vi "main(Test DQMH modules).vi"() -> ()   [LabVIEW 2018, in "Application.lvlib"] (continued)
          frame condition #0 (active) {
            n3006 = Empty String/Path?(string/path=w7173) -> (empty?=w7175:bool)
            n3007 = Select(t="Quece timeout", s=w7175, f=w7173) -> (s? t:f=w7172:string)
            n3008 = call "string log (SubVI).vi"("state Name"=w7172) -> ()  [unwired: 9 in, 2 out]
          }
          frame condition #1 {
          }
        }
        n3009 = Bundle By Name(cluster=w7125, "command"="Apps.UI Update", "data"="E") -> (w7124:T9)
        n3010 = Bundle By Name(cluster=w7125, "command"="MEAS.AllRelaysOFF2") -> (w7117:T9)
        n3011 = Bundle By Name(cluster=w7125, "command"="Apps.WaitForEvent") -> (w7123:T9)
        n3012 = Build Array(w7124, w7117, w7123) -> (w7130:T9[])
        n3013 = for {
          tunnel: [w7163] -> w7136 mode=indexing
          shift-right: [w7164] -> w7138
          shift-left: w7131 -> [w7162]
          tunnel: w7130 -> [w7161] mode=indexing
          n3014 = Unbundle By Name(w7161) -> ("command"=w7160:string, "data"=w7159:variant)
          n3015 = call "App enquece.vi"("Priority Enquece"=TRUE, "command data"=w7159, "command"=w7160, "queue in"=w7162) -> ("error out"=w7163:errorcluster, "Queue out"=w7164:refnum<queue>)  [unwired: 6 in]
        }
        n3016 = call "FGV DRV stand.vi"() -> ("Sub-Test.DCV"=w7118:bool)  [unwired: 10 in, 1 out]
        n3017 = case shown="True" w7118 {
          tunnel: [w7149 w7151] -> w7120
          frame False {
            n3018 = Build Array("WaitFor", "MEAS.requestAC") -> (w7149:string[])
          }
          frame True {
            n3019 = Build Array("Test DRV 31", "Test DRV 32", "Test DRV 33", "Test DRV 34", "Test DRV 35", "WaitForE", "MEAS.requestAC") -> (w7151:string[])
          }
        }
        n3020 = Merge Errors(w7136) -> (w7129:errorcluster)
        n3021 = Reverse 1D Array(array=w7120) -> (reversed array=w7116:string[])
        n3022 = for {
          tunnel: w7116 -> [w7170] mode=indexing
          tunnel: [w7169] -> w7135 mode=indexing
          shift-right: [w7168] -> w7137
          shift-left: w7138 -> [w7171]
          tunnel: w7129 -> [w7167]
          n3023 = call "App enquece.vi"("Priority Enquece"=TRUE, "error in (no error)"=w7167, "command"=w7170, "queue in"=w7171) -> ("error out"=w7169:errorcluster, "Queue out"=w7168:refnum<queue>)  [unwired: 6 in]
        }
        n3024 = Initialize Array(FALSE ("element"), 6 ("dimension size")) -> (w7099:bool[])
        n3025 = Initialize Array(TRUE, 5 ("dimension size")) -> (w7098:bool[])
        n3026 = Merge Errors(w7135) -> (w7134:errorcluster)
        n3027 = Replace Array Subset(array=w7099, new element=w7098) -> (w7097:bool[])  [unwired: 1 in]
        n3028 = To Variant(anything=T3."mux10_1_channel6" ("mux10_1(x6)_encode")) -> (Variant=w7114:variant)
        n3029 = To Variant(anything=T4."demux1_10_channel6" ("demux1_10(x6)_encode")) -> (Variant=w7110:variant)
        n3030 = To Variant(anything=w7097) -> (Variant=w7106:variant)
        n3031 = Bundle By Name(cluster=w7103, "command"="MEAS.mux10-1", "data"=w7114) -> (w7109:T9)
        n3032 = Bundle By Name(cluster=w7103, "command"="MEAS.demux1-10", "data"=w7110) -> (w7108:T9)
        n3033 = Bundle By Name(cluster=w7103, "command"="MEAS.eMIC", "data"=w7106) -> (w7105:T9)
        n3034 = Build Array(w7109, w7108, w7105) -> (w7133:T9[])
        n3035 = Reverse 1D Array(array=w7133) -> (reversed array=w7132:T9[])
        n3036 = for {
          tunnel: w7132 -> [w7181] mode=indexing
          tunnel: [w7178] -> w7139 mode=indexing
          tunnel: w7134 -> [w7177]
          tunnel: w7137 -> [w7182]
          n3037 = Unbundle By Name(w7181) -> ("command"=w7180:string, "data"=w7179:variant)
          n3038 = call "App enquece.vi"("Priority Enquece"=TRUE, "error in (no error)"=w7177, "command data"=w7179, "command"=w7180, "queue in"=w7182) -> ("error out"=w7178:errorcluster)  [unwired: 5 in, 1 out]
        }
        n3039 = Merge Errors(w7142, w7139) -> (w7143:errorcluster)
      }
      frame "Test Channel 7E" {
        w7189 = T9 {"command"="", "data"=variant} ("element")
        w7212 = T9 {"command"="", "data"=variant} ("element")
        w7231 = 7  # DUT channel (1-10)
        n3040 = disable-structure shown="LOGGING==TRUE" {
          disable-tunnel: w7226 -> [w7259 _]
          frame condition #0 (active) {
            n3041 = Empty String/Path?(string/path=w7259) -> (empty?=w7261:bool)
            n3042 = Select(t="Quece timeout", s=w7261, f=w7259) -> (s? t:f=w7258:string)
            n3043 = call "string log (SubVI).vi"("state Name"=w7258) -> ()  [unwired: 9 in, 2 out]
          }
          frame condition #1 {
          }
        }
        n3044 = Bundle By Name(cluster=w7212, "command"="Apps.UI Update", "data"="E") -> (w7211:T9)
        n3045 = Bundle By Name(cluster=w7212, "command"="MEAS.AllRelaysOFF2") -> (w7204:T9)
        n3046 = Bundle By Name(cluster=w7212, "command"="Apps.WaitForEvent") -> (w7210:T9)
        n3047 = Build Array(w7211, w7204, w7210) -> (w7202:T9[])
        n3048 = for {
          tunnel: [w7249] -> w7222 mode=indexing
          shift-right: [w7250] -> w7224
          shift-left: w7217 -> [w7248]
          tunnel: w7202 -> [w7247] mode=indexing
          n3049 = Unbundle By Name(w7247) -> ("command"=w7246:string, "data"=w7245:variant)
          n3050 = call "App enquece.vi"("Priority Enquece"=TRUE, "command data"=w7245, "command"=w7246, "queue in"=w7248) -> ("error out"=w7249:errorcluster, "Queue out"=w7250:refnum<queue>)  [unwired: 6 in]
        }
        n3051 = call "FGV DRV stand.vi"() -> ("Sub-Test.DCV"=w7205:bool)  [unwired: 10 in, 1 out]
        n3052 = case shown="True" w7205 {
          tunnel: [w7235 w7237] -> w7207
          frame False {
            n3053 = Build Array("WaitFor", "MEAS.requestAC") -> (w7235:string[])
          }
          frame True {
            n3054 = Build Array("Test DRV 37", "Test DRV 38", "Test DRV 39", "Test DRV 40", "Test DRV 41", "WaitForE", "MEAS.requestAC") -> (w7237:string[])
          }
        }
        n3055 = Merge Errors(w7222) -> (w7216:errorcluster)
        n3056 = Reverse 1D Array(array=w7207) -> (reversed array=w7203:string[])
        n3057 = for {
          tunnel: w7203 -> [w7256] mode=indexing
          tunnel: [w7255] -> w7221 mode=indexing
          shift-right: [w7254] -> w7223
          shift-left: w7224 -> [w7257]
          tunnel: w7216 -> [w7253]
          n3058 = call "App enquece.vi"("Priority Enquece"=TRUE, "error in (no error)"=w7253, "command"=w7256, "queue in"=w7257) -> ("error out"=w7255:errorcluster, "Queue out"=w7254:refnum<queue>)  [unwired: 6 in]
        }
        n3059 = Initialize Array(FALSE ("element"), 6 ("dimension size")) -> (w7185:bool[])
        n3060 = Initialize Array(TRUE, 5 ("dimension size")) -> (w7184:bool[])
        n3061 = Merge Errors(w7221) -> (w7220:errorcluster)
        n3062 = Replace Array Subset(array=w7185, new element=w7184) -> (w7183:bool[])  [unwired: 1 in]
        n3063 = To Variant(anything=T3."mux10_1_channel7" ("mux10_1(x6)_encode")) -> (Variant=w7200:variant)
        n3064 = To Variant(anything=T4."demux1_10_channel7" ("demux1_10(x6)_encode")) -> (Variant=w7196:variant)
        n3065 = To Variant(anything=w7183) -> (Variant=w7192:variant)
        n3066 = Bundle By Name(cluster=w7189, "command"="MEAS.mux10-1", "data"=w7200) -> (w7195:T9)
        n3067 = Bundle By Name(cluster=w7189, "command"="MEAS.demux1-10", "data"=w7196) -> (w7194:T9)
        n3068 = Bundle By Name(cluster=w7189, "command"="MEAS.eMIC", "data"=w7192) -> (w7191:T9)
        n3069 = Build Array(w7195, w7194, w7191) -> (w7219:T9[])
        n3070 = Reverse 1D Array(array=w7219) -> (reversed array=w7218:T9[])
        n3071 = for {
          tunnel: w7218 -> [w7267] mode=indexing
          tunnel: [w7264] -> w7225 mode=indexing
          tunnel: w7220 -> [w7263]
          tunnel: w7223 -> [w7268]
          n3072 = Unbundle By Name(w7267) -> ("command"=w7266:string, "data"=w7265:variant)
          n3073 = call "App enquece.vi"("Priority Enquece"=TRUE, "error in (no error)"=w7263, "command data"=w7265, "command"=w7266, "queue in"=w7268) -> ("error out"=w7264:errorcluster)  [unwired: 5 in, 1 out]
        }
        n3074 = Merge Errors(w7228, w7225) -> (w7229:errorcluster)
      }
      frame "Test Channel 8E" {
        w7275 = T9 {"command"="", "data"=variant} ("element")
        w7297 = T9 {"command"="", "data"=variant} ("element")
        w7317 = 8  # DUT channel (1-10)
        n3075 = disable-structure shown="LOGGING==TRUE" {
          disable-tunnel: w7312 -> [w7345 _]
          frame condition #0 (active) {
            n3076 = Empty String/Path?(string/path=w7345) -> (empty?=w7347:bool)
            n3077 = Select(t="Quece timeout", s=w7347, f=w7345) -> (s? t:f=w7344:string)
            n3078 = call "string log (SubVI).vi"("state Name"=w7344) -> ()  [unwired: 9 in, 2 out]
          }
          frame condition #1 {
          }
        }
        n3079 = Bundle By Name(cluster=w7297, "command"="Apps.UI Update", "data"="E") -> (w7296:T9)
        n3080 = Bundle By Name(cluster=w7297, "command"="MEAS.AllRelaysOFF2") -> (w7289:T9)
        n3081 = Bundle By Name(cluster=w7297, "command"="Apps.WaitForEvent") -> (w7295:T9)
        n3082 = Build Array(w7296, w7289, w7295) -> (w7302:T9[])
        n3083 = for {
          tunnel: [w7335] -> w7308 mode=indexing
          shift-right: [w7336] -> w7310
          shift-left: w7303 -> [w7334]
          tunnel: w7302 -> [w7333] mode=indexing
          n3084 = Unbundle By Name(w7333) -> ("command"=w7332:string, "data"=w7331:variant)
          n3085 = call "App enquece.vi"("Priority Enquece"=TRUE, "command data"=w7331, "command"=w7332, "queue in"=w7334) -> ("error out"=w7335:errorcluster, "Queue out"=w7336:refnum<queue>)  [unwired: 6 in]
        }
        n3086 = call "FGV DRV stand.vi"() -> ("Sub-Test.DCV"=w7290:bool)  [unwired: 10 in, 1 out]
        n3087 = case shown="True" w7290 {
          tunnel: [w7321 w7323] -> w7292
          frame False {
            n3088 = Build Array("WaitFor", "MEAS.requestAC") -> (w7321:string[])
          }
          frame True {
            n3089 = Build Array("Test DRV 43", "Test DRV 44", "Test DRV 45", "Test DRV 46", "Test DRV 47", "WaitForE", "MEAS.requestAC") -> (w7323:string[])
          }
        }
        n3090 = Merge Errors(w7308) -> (w7301:errorcluster)
        n3091 = Reverse 1D Array(array=w7292) -> (reversed array=w7288:string[])
        n3092 = for {
          tunnel: w7288 -> [w7342] mode=indexing
          tunnel: [w7341] -> w7307 mode=indexing
          shift-right: [w7340] -> w7309
          shift-left: w7310 -> [w7343]
          tunnel: w7301 -> [w7339]
          n3093 = call "App enquece.vi"("Priority Enquece"=TRUE, "error in (no error)"=w7339, "command"=w7342, "queue in"=w7343) -> ("error out"=w7341:errorcluster, "Queue out"=w7340:refnum<queue>)  [unwired: 6 in]
        }
        n3094 = Initialize Array(FALSE ("element"), 6 ("dimension size")) -> (w7271:bool[])
        n3095 = Initialize Array(TRUE, 5 ("dimension size")) -> (w7270:bool[])
        n3096 = Merge Errors(w7307) -> (w7306:errorcluster)
        n3097 = Replace Array Subset(array=w7271, new element=w7270) -> (w7269:bool[])  [unwired: 1 in]
        n3098 = To Variant(anything=T3."mux10_1_channel8" ("mux10_1(x6)_encode")) -> (Variant=w7286:variant)
        n3099 = To Variant(anything=T4."demux1_10_channel8" ("demux1_10(x6)_encode")) -> (Variant=w7282:variant)
        n3100 = To Variant(anything=w7269) -> (Variant=w7278:variant)
        n3101 = Bundle By Name(cluster=w7275, "command"="MEAS.mux10-1", "data"=w7286) -> (w7281:T9)
        n3102 = Bundle By Name(cluster=w7275, "command"="MEAS.demux1-10", "data"=w7282) -> (w7280:T9)
        n3103 = Bundle By Name(cluster=w7275, "command"="MEAS.eMIC", "data"=w7278) -> (w7277:T9)
        n3104 = Build Array(w7281, w7280, w7277) -> (w7305:T9[])
        n3105 = Reverse 1D Array(array=w7305) -> (reversed array=w7304:T9[])
        n3106 = for {
          tunnel: w7304 -> [w7353] mode=indexing
          tunnel: [w7350] -> w7311 mode=indexing
          tunnel: w7306 -> [w7349]
          tunnel: w7309 -> [w7354]
          n3107 = Unbundle By Name(w7353) -> ("command"=w7352:string, "data"=w7351:variant)
          n3108 = call "App enquece.vi"("Priority Enquece"=TRUE, "error in (no error)"=w7349, "command data"=w7351, "command"=w7352, "queue in"=w7354) -> ("error out"=w7350:errorcluster)  [unwired: 5 in, 1 out]
        }
        n3109 = Merge Errors(w7314, w7311) -> (w7315:errorcluster)
      }
      frame "Test Channel 9E" {
        w7361 = T9 {"command"="", "data"=variant} ("element")
        w7383 = T9 {"command"="", "data"=variant} ("element")
        w7403 = 9  # DUT channel (1-10)
        n3110 = disable-structure shown="LOGGING==TRUE" {
          disable-tunnel: w7398 -> [w7431 _]
          frame condition #0 (active) {
            n3111 = Empty String/Path?(string/path=w7431) -> (empty?=w7433:bool)
            n3112 = Select(t="Quece timeout", s=w7433, f=w7431) -> (s? t:f=w7430:string)
            n3113 = call "string log (SubVI).vi"("state Name"=w7430) -> ()  [unwired: 9 in, 2 out]
          }
          frame condition #1 {
          }
        }
        n3114 = Bundle By Name(cluster=w7383, "command"="Apps.UI Update", "data"="E") -> (w7382:T9)
        n3115 = Bundle By Name(cluster=w7383, "command"="MEAS.AllRelaysOFF2") -> (w7375:T9)
        n3116 = Bundle By Name(cluster=w7383, "command"="Apps.WaitForEvent") -> (w7381:T9)
        n3117 = Build Array(w7382, w7375, w7381) -> (w7388:T9[])
        n3118 = for {
          tunnel: [w7421] -> w7394 mode=indexing
          shift-right: [w7422] -> w7396
          shift-left: w7389 -> [w7420]
          tunnel: w7388 -> [w7419] mode=indexing
          n3119 = Unbundle By Name(w7419) -> ("command"=w7418:string, "data"=w7417:variant)
          n3120 = call "App enquece.vi"("Priority Enquece"=TRUE, "command data"=w7417, "command"=w7418, "queue in"=w7420) -> ("error out"=w7421:errorcluster, "Queue out"=w7422:refnum<queue>)  [unwired: 6 in]
        }
        n3121 = call "FGV DRV stand.vi"() -> ("Sub-Test.DCV"=w7376:bool)  [unwired: 10 in, 1 out]
        n3122 = case shown="True" w7376 {
          tunnel: [w7407 w7409] -> w7378
          frame False {
            n3123 = Build Array("WaitFor", "MEAS.requestAC") -> (w7407:string[])
          }
          frame True {
            n3124 = Build Array("Test DRV 49", "Test DRV 50", "Test DRV 51", "Test DRV 52", "Test DRV 53", "WaitForE", "MEAS.requestAC") -> (w7409:string[])
          }
        }
        n3125 = Merge Errors(w7394) -> (w7387:errorcluster)
        n3126 = Reverse 1D Array(array=w7378) -> (reversed array=w7374:string[])
        n3127 = for {
          tunnel: w7374 -> [w7428] mode=indexing
          tunnel: [w7427] -> w7393 mode=indexing
          shift-right: [w7426] -> w7395
          shift-left: w7396 -> [w7429]
          tunnel: w7387 -> [w7425]
          n3128 = call "App enquece.vi"("Priority Enquece"=TRUE, "error in (no error)"=w7425, "command"=w7428, "queue in"=w7429) -> ("error out"=w7427:errorcluster, "Queue out"=w7426:refnum<queue>)  [unwired: 6 in]
        }
        n3129 = Merge Errors(w7393) -> (w7392:errorcluster)
        n3130 = Initialize Array(FALSE ("element"), 6 ("dimension size")) -> (w7357:bool[])
        n3131 = Initialize Array(TRUE, 5 ("dimension size")) -> (w7356:bool[])
        n3132 = Replace Array Subset(array=w7357, new element=w7356) -> (w7355:bool[])  [unwired: 1 in]
        n3133 = To Variant(anything=T3."mux10_1_channel9" ("mux10_1(x6)_encode")) -> (Variant=w7372:variant)
        n3134 = To Variant(anything=T4."demux1_10_channel9" ("demux1_10(x6)_encode")) -> (Variant=w7368:variant)
        n3135 = To Variant(anything=w7355) -> (Variant=w7364:variant)
        n3136 = Bundle By Name(cluster=w7361, "command"="MEAS.mux10-1", "data"=w7372) -> (w7367:T9)
        n3137 = Bundle By Name(cluster=w7361, "command"="MEAS.demux1-10", "data"=w7368) -> (w7366:T9)
        n3138 = Bundle By Name(cluster=w7361, "command"="MEAS.eMIC", "data"=w7364) -> (w7363:T9)
        n3139 = Build Array(w7367, w7366, w7363) -> (w7391:T9[])
        n3140 = Reverse 1D Array(array=w7391) -> (reversed array=w7390:T9[])
        n3141 = for {
          tunnel: w7390 -> [w7439] mode=indexing
          tunnel: [w7436] -> w7397 mode=indexing
          tunnel: w7392 -> [w7435]
          tunnel: w7395 -> [w7440]
          n3142 = Unbundle By Name(w7439) -> ("command"=w7438:string, "data"=w7437:variant)
          n3143 = call "App enquece.vi"("Priority Enquece"=TRUE, "error in (no error)"=w7435, "command data"=w7437, "command"=w7438, "queue in"=w7440) -> ("error out"=w7436:errorcluster)  [unwired: 5 in, 1 out]
        }
        n3144 = Merge Errors(w7400, w7397) -> (w7401:errorcluster)
      }
      frame "Test DRV 1" {
        w7445 = 1  # DUT index(1-60)
        n3145 = disable-structure shown="LOGGING==TRUE" {
          disable-tunnel: w7448 -> [w7479 _]
          frame condition #0 (active) {
            n3146 = Empty String/Path?(string/path=w7479) -> (empty?=w7481:bool)
            n3147 = Select(t="Quece timeout", s=w7481, f=w7479) -> (s? t:f=w7478:string)
            n3148 = call "string log (SubVI).vi"("state Name"=w7478) -> ()  [unwired: 9 in, 2 out]
          }
          frame condition #1 {
          }
        }
        n3149 = call "progress string(SubVI).vi"("String 3"=w7448, "String in"=w7446) -> ("String out"=w7447:string)  [unwired: 9 in]
        n3150 = call "FGV DRV stand.vi"() -> ("Sub-Test.DCV"=w7444:bool)  [unwired: 10 in, 1 out]
        n3151 = call "FGV Driver Data.vi"("DUT index(1-60)"=w7445) -> ("DUT SC"=w7443:bool)  [unwired: 7 in, 3 out]
        n3152 = Not(x=w7444) -> (.not. x?=w7441:bool)
        n3153 = Or(x=w7443, y=w7441) -> (x .or. y?=w7442:bool)
        n3154 = case shown="False" w7442 {
          tunnel: [w7471 _] -> w7453
          tunnel: w7450 -> [w7470 _]
          frame False {
            w7459 = T9 {"command"="", "data"=variant} ("element")
            w7458 = "MEAS.mux6_1"
            n3155 = To Variant(anything=T2."mux6_1_channel1_3" ("mux6_1(3wires)_encode")) -> (Variant=w7468:variant)
            n3156 = To Variant(anything=T2."mux6-1_channel1_2" ("mux6_1(3wires)_encode")) -> (Variant=w7466:variant)
            n3157 = Bundle By Name(cluster=w7459, "command"=w7458, "data"=w7466) -> (w7465:T9)
            n3158 = Bundle By Name(cluster=w7459, "command"=w7458, "data"=w7468) -> (w7464:T9)
            n3159 = Bundle By Name(cluster=w7459, "command"="MEAS.DMM dual read") -> (w7462:T9)
            n3160 = Build Array(w7465, w7464, w7462) -> (w7460:T9[])
            n3161 = Reverse 1D Array(array=w7460) -> (reversed array=w7461:T9[])
            n3162 = for {
              tunnel: [w7477] -> w7471 mode=indexing
              tunnel: w7470 -> [w7476]
              tunnel: w7461 -> [w7475] mode=indexing
              n3163 = Unbundle By Name(w7475) -> ("command"=w7474:string, "data"=w7473:variant)
              n3164 = call "App enquece.vi"("Priority Enquece"=TRUE, "command data"=w7473, "command"=w7474, "queue in"=w7476) -> ("error out"=w7477:errorcluster)  [unwired: 6 in, 1 out]
            }
          }
          frame True {
          }
        }
        n3165 = Merge Errors(w7451, w7453) -> (w7452:errorcluster)
      }
      frame "Test DRV 2" {
        w7487 = 2  # DUT index(1-60)
        n3166 = disable-structure shown="LOGGING==TRUE" {
          disable-tunnel: w7488 -> [w7520 _]
          frame condition #0 (active) {
            n3167 = Empty String/Path?(string/path=w7520) -> (empty?=w7522:bool)
            n3168 = Select(t="Quece timeout", s=w7522, f=w7520) -> (s? t:f=w7519:string)
            n3169 = call "string log (SubVI).vi"("state Name"=w7519) -> ()  [unwired: 9 in, 2 out]
          }
          frame condition #1 {
          }
        }
        n3170 = call "progress string(SubVI).vi"("String 3"=w7488, "String in"=w7489) -> ("String out"=w7490:string)  [unwired: 9 in]
        n3171 = call "FGV DRV stand.vi"() -> ("Sub-Test.DCV"=w7486:bool)  [unwired: 10 in, 1 out]
        n3172 = call "FGV Driver Data.vi"("DUT index(1-60)"=w7487) -> ("DUT SC"=w7485:bool)  [unwired: 7 in, 3 out]
        n3173 = Not(x=w7486) -> (.not. x?=w7483:bool)
        n3174 = Or(x=w7485, y=w7483) -> (x .or. y?=w7484:bool)
        n3175 = case shown="False" w7484 {
          tunnel: [w7512 _] -> w7494
          tunnel: w7492 -> [w7511 _]
          frame False {
            w7499 = T9 {"command"="", "data"=variant} ("element")
            w7500 = "MEAS.mux6_1"
            n3176 = To Variant(anything=T2."mux6_1_channel2_3" ("mux6_1(3wires)_encode")) -> (Variant=w7509:variant)
            n3177 = To Variant(anything=T2."mux6_1_channel2_2" ("mux6_1(3wires)_encode")) -> (Variant=w7507:variant)
            n3178 = Bundle By Name(cluster=w7499, "command"=w7500, "data"=w7507) -> (w7506:T9)
            n3179 = Bundle By Name(cluster=w7499, "command"=w7500, "data"=w7509) -> (w7505:T9)
            n3180 = Bundle By Name(cluster=w7499, "command"="MEAS.DMM dual read") -> (w7503:T9)
            n3181 = Build Array(w7506, w7505, w7503) -> (w7501:T9[])
            n3182 = Reverse 1D Array(array=w7501) -> (reversed array=w7502:T9[])
            n3183 = for {
              tunnel: [w7518] -> w7512 mode=indexing
              tunnel: w7511 -> [w7517]
              tunnel: w7502 -> [w7516] mode=indexing
              n3184 = Unbundle By Name(w7516) -> ("command"=w7515:string, "data"=w7514:variant)
              n3185 = call "App enquece.vi"("Priority Enquece"=TRUE, "command data"=w7514, "command"=w7515, "queue in"=w7517) -> ("error out"=w7518:errorcluster)  [unwired: 6 in, 1 out]
            }
          }
          frame True {
          }
        }
        n3186 = Merge Errors(w7493, w7494) -> (w7482:errorcluster)
      }
      frame "Test DRV 3" {
        w7527 = 3  # DUT index(1-60)
        n3187 = disable-structure shown="LOGGING==TRUE" {
          disable-tunnel: w7528 -> [w7561 _]
          frame condition #0 (active) {
            n3188 = Empty String/Path?(string/path=w7561) -> (empty?=w7563:bool)
            n3189 = Select(t="Quece timeout", s=w7563, f=w7561) -> (s? t:f=w7560:string)
            n3190 = call "string log (SubVI).vi"("state Name"=w7560) -> ()  [unwired: 9 in, 2 out]
          }
          frame condition #1 {
          }
        }
        n3191 = call "progress string(SubVI).vi"("String 3"=w7528, "String in"=w7529) -> ("String out"=w7530:string)  [unwired: 9 in]
        n3192 = call "FGV DRV stand.vi"() -> ("Sub-Test.DCV"=w7526:bool)  [unwired: 10 in, 1 out]
        n3193 = call "FGV Driver Data.vi"("DUT index(1-60)"=w7527) -> ("DUT SC"=w7525:bool)  [unwired: 7 in, 3 out]
        n3194 = Not(x=w7526) -> (.not. x?=w7523:bool)
        n3195 = Or(x=w7525, y=w7523) -> (x .or. y?=w7524:bool)
        n3196 = case shown="True" w7524 {
          tunnel: [w7553 _] -> w7535
          tunnel: w7532 -> [w7552 _]
          frame False {
            w7541 = T9 {"command"="", "data"=variant} ("element")
            w7540 = "MEAS.mux6_1"
            n3197 = To Variant(anything=T2."mux6_1_channel3_3" ("mux6_1(3wires)_encode")) -> (Variant=w7550:variant)
            n3198 = To Variant(anything=T2."mux6_1_channel3_2" ("mux6_1(3wires)_encode")) -> (Variant=w7548:variant)
            n3199 = Bundle By Name(cluster=w7541, "command"=w7540, "data"=w7548) -> (w7547:T9)
            n3200 = Bundle By Name(cluster=w7541, "command"=w7540, "data"=w7550) -> (w7546:T9)
            n3201 = Bundle By Name(cluster=w7541, "command"="MEAS.DMM dual read") -> (w7544:T9)
            n3202 = Build Array(w7547, w7546, w7544) -> (w7542:T9[])
            n3203 = Reverse 1D Array(array=w7542) -> (reversed array=w7543:T9[])
            n3204 = for {
              tunnel: [w7559] -> w7553 mode=indexing
              tunnel: w7552 -> [w7558]
              tunnel: w7543 -> [w7557] mode=indexing
              n3205 = Unbundle By Name(w7557) -> ("command"=w7556:string, "data"=w7555:variant)
              n3206 = call "App enquece.vi"("Priority Enquece"=TRUE, "command data"=w7555, "command"=w7556, "queue in"=w7558) -> ("error out"=w7559:errorcluster)  [unwired: 6 in, 1 out]
            }
          }
          frame True {
          }
        }
        n3207 = Merge Errors(w7533, w7535) -> (w7534:errorcluster)
      }
      frame "Test DRV 4" {
        w7568 = 4  # DUT index(1-60)
        n3208 = disable-structure shown="LOGGING==TRUE" {
          disable-tunnel: w7569 -> [w7601 _]
          frame condition #0 (active) {
            n3209 = Empty String/Path?(string/path=w7601) -> (empty?=w7604:bool)
            n3210 = Select(t="Quece timeout", s=w7604, f=w7601) -> (s? t:f=w7602:string)
            n3211 = call "string log (SubVI).vi"("state Name"=w7602) -> ()  [unwired: 9 in, 2 out]
          }
          frame condition #1 {
          }
        }
        n3212 = call "progress string(SubVI).vi"("String 3"=w7569, "String in"=w7570) -> ("String out"=w7571:string)  [unwired: 9 in]
        n3213 = call "FGV DRV stand.vi"() -> ("Sub-Test.DCV"=w7567:bool)  [unwired: 10 in, 1 out]
        n3214 = call "FGV Driver Data.vi"("DUT index(1-60)"=w7568) -> ("DUT SC"=w7566:bool)  [unwired: 7 in, 3 out]
        n3215 = Not(x=w7567) -> (.not. x?=w7564:bool)
        n3216 = Or(x=w7566, y=w7564) -> (x .or. y?=w7565:bool)
        n3217 = case shown="False" w7565 {
          tunnel: [w7594 _] -> w7576
          tunnel: w7573 -> [w7593 _]
          frame False {
            w7582 = T9 {"command"="", "data"=variant} ("element")
            w7581 = "MEAS.mux6_1"
            n3218 = To Variant(anything=T2."mux6_1_channel4_3" ("mux6_1(3wires)_encode")) -> (Variant=w7591:variant)
            n3219 = To Variant(anything=T2."mux6_1_channel4_2" ("mux6_1(3wires)_encode")) -> (Variant=w7589:variant)
            n3220 = Bundle By Name(cluster=w7582, "command"=w7581, "data"=w7589) -> (w7588:T9)
            n3221 = Bundle By Name(cluster=w7582, "command"=w7581, "data"=w7591) -> (w7587:T9)
            n3222 = Bundle By Name(cluster=w7582, "command"="MEAS.DMM dual read") -> (w7585:T9)
            n3223 = Build Array(w7588, w7587, w7585) -> (w7583:T9[])
            n3224 = Reverse 1D Array(array=w7583) -> (reversed array=w7584:T9[])
            n3225 = for {
              tunnel: [w7600] -> w7594 mode=indexing
              tunnel: w7593 -> [w7599]
              tunnel: w7584 -> [w7598] mode=indexing
              n3226 = Unbundle By Name(w7598) -> ("command"=w7597:string, "data"=w7596:variant)
              n3227 = call "App enquece.vi"("Priority Enquece"=TRUE, "command data"=w7596, "command"=w7597, "queue in"=w7599) -> ("error out"=w7600:errorcluster)  [unwired: 6 in, 1 out]
            }
          }
          frame True {
          }
        }
        n3228 = Merge Errors(w7574, w7576) -> (w7575:errorcluster)
      }
      frame "Test DRV 5" {
        w7609 = 5  # DUT index(1-60)
        n3229 = disable-structure shown="LOGGING==TRUE" {
          disable-tunnel: w7610 -> [w7643 _]
          frame condition #0 (active) {
            n3230 = Empty String/Path?(string/path=w7643) -> (empty?=w7645:bool)
            n3231 = Select(t="Quece timeout", s=w7645, f=w7643) -> (s? t:f=w7642:string)
            n3232 = call "string log (SubVI).vi"("state Name"=w7642) -> ()  [unwired: 9 in, 2 out]
          }
          frame condition #1 {
          }
        }
        n3233 = call "progress string(SubVI).vi"("String 3"=w7610, "String in"=w7611) -> ("String out"=w7612:string)  [unwired: 9 in]
        n3234 = call "FGV DRV stand.vi"() -> ("Sub-Test.DCV"=w7608:bool)  [unwired: 10 in, 1 out]
        n3235 = call "FGV Driver Data.vi"("DUT index(1-60)"=w7609) -> ("DUT SC"=w7607:bool)  [unwired: 7 in, 3 out]
        n3236 = Not(x=w7608) -> (.not. x?=w7605:bool)
        n3237 = Or(x=w7607, y=w7605) -> (x .or. y?=w7606:bool)
        n3238 = case shown="False" w7606 {
          tunnel: [w7635 _] -> w7617
          tunnel: w7614 -> [w7634 _]
          frame False {
            w7623 = T9 {"command"="", "data"=variant} ("element")
            w7622 = "MEAS.mux6_1"
            n3239 = To Variant(anything=T2."mux6_1_channel5_3" ("mux6_1(3wires)_encode")) -> (Variant=w7632:variant)
            n3240 = To Variant(anything=T2."mux6_1_channel5_2" ("mux6_1(3wires)_encode")) -> (Variant=w7630:variant)
            n3241 = Bundle By Name(cluster=w7623, "command"=w7622, "data"=w7630) -> (w7629:T9)
            n3242 = Bundle By Name(cluster=w7623, "command"=w7622, "data"=w7632) -> (w7628:T9)
            n3243 = Bundle By Name(cluster=w7623, "command"="MEAS.DMM dual read") -> (w7626:T9)
            n3244 = Build Array(w7629, w7628, w7626) -> (w7624:T9[])
            n3245 = Reverse 1D Array(array=w7624) -> (reversed array=w7625:T9[])
            n3246 = for {
              tunnel: [w7641] -> w7635 mode=indexing
              tunnel: w7634 -> [w7640]
              tunnel: w7625 -> [w7639] mode=indexing
              n3247 = Unbundle By Name(w7639) -> ("command"=w7638:string, "data"=w7637:variant)
              n3248 = call "App enquece.vi"("Priority Enquece"=TRUE, "command data"=w7637, "command"=w7638, "queue in"=w7640) -> ("error out"=w7641:errorcluster)  [unwired: 6 in, 1 out]
            }
          }
          frame True {
          }
        }
        n3249 = Merge Errors(w7615, w7617) -> (w7616:errorcluster)
      }
      frame "Test DRV 6" {
        w7653 = 6  # DUT index(1-60)
        n3250 = disable-structure shown="LOGGING==TRUE" {
          disable-tunnel: w7650 -> [w7684 _]
          frame condition #0 (active) {
            n3251 = Empty String/Path?(string/path=w7684) -> (empty?=w7686:bool)
            n3252 = Select(t="Quece timeout", s=w7686, f=w7684) -> (s? t:f=w7683:string)
            n3253 = call "string log (SubVI).vi"("state Name"=w7683) -> ()  [unwired: 9 in, 2 out]
          }
          frame condition #1 {
          }
        }
        n3254 = call "progress string(SubVI).vi"("String 3"=w7650, "String in"=w7651) -> ("String out"=w7652:string)  [unwired: 9 in]
        n3255 = call "FGV DRV stand.vi"() -> ("Sub-Test.DCV"=w7649:bool)  [unwired: 10 in, 1 out]
        n3256 = call "FGV Driver Data.vi"("DUT index(1-60)"=w7653) -> ("DUT SC"=w7648:bool)  [unwired: 7 in, 3 out]
        n3257 = Not(x=w7649) -> (.not. x?=w7646:bool)
        n3258 = Or(x=w7648, y=w7646) -> (x .or. y?=w7647:bool)
        n3259 = case shown="False" w7647 {
          tunnel: [w7676 _] -> w7658
          tunnel: w7655 -> [w7675 _]
          frame False {
            w7664 = T9 {"command"="", "data"=variant} ("element")
            w7663 = "MEAS.mux6_1"
            n3260 = To Variant(anything=T2."mux6_1_channel6_3" ("mux6_1(3wires)_encode")) -> (Variant=w7673:variant)
            n3261 = To Variant(anything=T2."mux6_1_channel6_2" ("mux6_1(3wires)_encode")) -> (Variant=w7671:variant)
            n3262 = Bundle By Name(cluster=w7664, "command"=w7663, "data"=w7671) -> (w7670:T9)
            n3263 = Bundle By Name(cluster=w7664, "command"=w7663, "data"=w7673) -> (w7669:T9)
            n3264 = Bundle By Name(cluster=w7664, "command"="MEAS.DMM dual read") -> (w7667:T9)
            n3265 = Build Array(w7670, w7669, w7667) -> (w7665:T9[])
            n3266 = Reverse 1D Array(array=w7665) -> (reversed array=w7666:T9[])
            n3267 = for {
              tunnel: [w7682] -> w7676 mode=indexing
              tunnel: w7675 -> [w7681]
              tunnel: w7666 -> [w7680] mode=indexing
              n3268 = Unbundle By Name(w7680) -> ("command"=w7679:string, "data"=w7678:variant)
              n3269 = call "App enquece.vi"("Priority Enquece"=TRUE, "command data"=w7678, "command"=w7679, "queue in"=w7681) -> ("error out"=w7682:errorcluster)  [unwired: 6 in, 1 out]
            }
          }
          frame True {
          }
        }
        n3270 = Merge Errors(w7656, w7658) -> (w7657:errorcluster)
      }
      frame "Test DRV 7" {
        w7691 = 7  # DUT index(1-60)
        n3271 = disable-structure shown="LOGGING==TRUE" {
          disable-tunnel: w7692 -> [w7725 _]
          frame condition #0 (active) {
            n3272 = Empty String/Path?(string/path=w7725) -> (empty?=w7727:bool)
            n3273 = Select(t="Quece timeout", s=w7727, f=w7725) -> (s? t:f=w7724:string)
            n3274 = call "string log (SubVI).vi"("state Name"=w7724) -> ()  [unwired: 9 in, 2 out]
          }
          frame condition #1 {
          }
        }
        n3275 = call "progress string(SubVI).vi"("String 3"=w7692, "String in"=w7693) -> ("String out"=w7694:string)  [unwired: 9 in]
        n3276 = call "FGV DRV stand.vi"() -> ("Sub-Test.DCV"=w7690:bool)  [unwired: 10 in, 1 out]
        n3277 = call "FGV Driver Data.vi"("DUT index(1-60)"=w7691) -> ("DUT SC"=w7689:bool)  [unwired: 7 in, 3 out]
        n3278 = Not(x=w7690) -> (.not. x?=w7687:bool)
        n3279 = Or(x=w7689, y=w7687) -> (x .or. y?=w7688:bool)
        n3280 = case shown="False" w7688 {
          tunnel: [w7717 _] -> w7699
          tunnel: w7696 -> [w7716 _]
          frame False {
            w7705 = T9 {"command"="", "data"=variant} ("element")
            w7704 = "MEAS.mux6_1"
            n3281 = To Variant(anything=T2."mux6_1_channel1_3" ("mux6_1(3wires)_encode")) -> (Variant=w7714:variant)
            n3282 = To Variant(anything=T2."mux6-1_channel1_2" ("mux6_1(3wires)_encode")) -> (Variant=w7712:variant)
            n3283 = Bundle By Name(cluster=w7705, "command"=w7704, "data"=w7712) -> (w7711:T9)
            n3284 = Bundle By Name(cluster=w7705, "command"=w7704, "data"=w7714) -> (w7710:T9)
            n3285 = Bundle By Name(cluster=w7705, "command"="MEAS.DMM dual read") -> (w7708:T9)
            n3286 = Build Array(w7711, w7710, w7708) -> (w7706:T9[])
            n3287 = Reverse 1D Array(array=w7706) -> (reversed array=w7707:T9[])
            n3288 = for {
              tunnel: [w7723] -> w7717 mode=indexing
              tunnel: w7716 -> [w7722]
              tunnel: w7707 -> [w7721] mode=indexing
              n3289 = Unbundle By Name(w7721) -> ("command"=w7720:string, "data"=w7719:variant)
              n3290 = call "App enquece.vi"("Priority Enquece"=TRUE, "command data"=w7719, "command"=w7720, "queue in"=w7722) -> ("error out"=w7723:errorcluster)  [unwired: 6 in, 1 out]
            }
          }
          frame True {
          }
        }
        n3291 = Merge Errors(w7697, w7699) -> (w7698:errorcluster)
      }
      frame "Test DRV 8" {
        w7732 = 8  # DUT index(1-60)
        n3292 = disable-structure shown="LOGGING==TRUE" {
          disable-tunnel: w7733 -> [w7766 _]
          frame condition #0 (active) {
            n3293 = Empty String/Path?(string/path=w7766) -> (empty?=w7768:bool)
            n3294 = Select(t="Quece timeout", s=w7768, f=w7766) -> (s? t:f=w7765:string)
            n3295 = call "string log (SubVI).vi"("state Name"=w7765) -> ()  [unwired: 9 in, 2 out]
          }
          frame condition #1 {
          }
        }
        n3296 = call "progress string(SubVI).vi"("String 3"=w7733, "String in"=w7734) -> ("String out"=w7735:string)  [unwired: 9 in]
        n3297 = call "FGV DRV stand.vi"() -> ("Sub-Test.DCV"=w7731:bool)  [unwired: 10 in, 1 out]
        n3298 = call "FGV Driver Data.vi"("DUT index(1-60)"=w7732) -> ("DUT SC"=w7730:bool)  [unwired: 7 in, 3 out]
        n3299 = Not(x=w7731) -> (.not. x?=w7728:bool)
        n3300 = Or(x=w7730, y=w7728) -> (x .or. y?=w7729:bool)
        n3301 = case shown="False" w7729 {
          tunnel: [w7758 _] -> w7740
          tunnel: w7737 -> [w7757 _]
          frame False {
            w7746 = T9 {"command"="", "data"=variant} ("element")
            w7745 = "MEAS.mux6_1"
            n3302 = To Variant(anything=T2."mux6_1_channel2_3" ("mux6_1(3wires)_encode")) -> (Variant=w7755:variant)
            n3303 = To Variant(anything=T2."mux6_1_channel2_2" ("mux6_1(3wires)_encode")) -> (Variant=w7753:variant)
            n3304 = Bundle By Name(cluster=w7746, "command"=w7745, "data"=w7753) -> (w7752:T9)
            n3305 = Bundle By Name(cluster=w7746, "command"=w7745, "data"=w7755) -> (w7751:T9)
            n3306 = Bundle By Name(cluster=w7746, "command"="MEAS.DMM dual read") -> (w7749:T9)
            n3307 = Build Array(w7752, w7751, w7749) -> (w7747:T9[])
            n3308 = Reverse 1D Array(array=w7747) -> (reversed array=w7748:T9[])
            n3309 = for {
              tunnel: [w7764] -> w7758 mode=indexing
              tunnel: w7757 -> [w7763]
              tunnel: w7748 -> [w7762] mode=indexing
              n3310 = Unbundle By Name(w7762) -> ("command"=w7761:string, "data"=w7760:variant)
              n3311 = call "App enquece.vi"("Priority Enquece"=TRUE, "command data"=w7760, "command"=w7761, "queue in"=w7763) -> ("error out"=w7764:errorcluster)  [unwired: 6 in, 1 out]
            }
          }
          frame True {
          }
        }
        n3312 = Merge Errors(w7738, w7740) -> (w7739:errorcluster)
      }
      frame "Test DRV 9" {
        w7773 = 9  # DUT index(1-60)
        n3313 = disable-structure shown="LOGGING==TRUE" {
          disable-tunnel: w7774 -> [w7807 _]
          frame condition #0 (active) {
            n3314 = Empty String/Path?(string/path=w7807) -> (empty?=w7809:bool)
            n3315 = Select(t="Quece timeout", s=w7809, f=w7807) -> (s? t:f=w7806:string)
            n3316 = call "string log (SubVI).vi"("state Name"=w7806) -> ()  [unwired: 9 in, 2 out]
          }
          frame condition #1 {
          }
        }
        n3317 = call "progress string(SubVI).vi"("String 3"=w7774, "String in"=w7775) -> ("String out"=w7776:string)  [unwired: 9 in]
        n3318 = call "FGV DRV stand.vi"() -> ("Sub-Test.DCV"=w7772:bool)  [unwired: 10 in, 1 out]
        n3319 = call "FGV Driver Data.vi"("DUT index(1-60)"=w7773) -> ("DUT SC"=w7771:bool)  [unwired: 7 in, 3 out]
        n3320 = Not(x=w7772) -> (.not. x?=w7769:bool)
        n3321 = Or(x=w7771, y=w7769) -> (x .or. y?=w7770:bool)
        n3322 = case shown="False" w7770 {
          tunnel: [w7799 _] -> w7781
          tunnel: w7778 -> [w7798 _]
          frame False {
            w7787 = T9 {"command"="", "data"=variant} ("element")
            w7786 = "MEAS.mux6_1"
            n3323 = To Variant(anything=T2."mux6_1_channel3_3" ("mux6_1(3wires)_encode")) -> (Variant=w7796:variant)
            n3324 = To Variant(anything=T2."mux6_1_channel3_2" ("mux6_1(3wires)_encode")) -> (Variant=w7794:variant)
            n3325 = Bundle By Name(cluster=w7787, "command"=w7786, "data"=w7794) -> (w7793:T9)
            n3326 = Bundle By Name(cluster=w7787, "command"=w7786, "data"=w7796) -> (w7792:T9)
            n3327 = Bundle By Name(cluster=w7787, "command"="MEAS.DMM dual read") -> (w7790:T9)
            n3328 = Build Array(w7793, w7792, w7790) -> (w7788:T9[])
            n3329 = Reverse 1D Array(array=w7788) -> (reversed array=w7789:T9[])
            n3330 = for {
              tunnel: [w7805] -> w7799 mode=indexing
              tunnel: w7798 -> [w7804]
              tunnel: w7789 -> [w7803] mode=indexing
              n3331 = Unbundle By Name(w7803) -> ("command"=w7802:string, "data"=w7801:variant)
              n3332 = call "App enquece.vi"("Priority Enquece"=TRUE, "command data"=w7801, "command"=w7802, "queue in"=w7804) -> ("error out"=w7805:errorcluster)  [unwired: 6 in, 1 out]
            }
          }
          frame True {
          }
        }
        n3333 = Merge Errors(w7779, w7781) -> (w7780:errorcluster)
      }
      frame "Test DRV 10" {
        w7814 = 10  # DUT index(1-60)
        n3334 = disable-structure shown="LOGGING==TRUE" {
          disable-tunnel: w7815 -> [w7848 _]
          frame condition #0 (active) {
            n3335 = Empty String/Path?(string/path=w7848) -> (empty?=w7850:bool)
            n3336 = Select(t="Quece timeout", s=w7850, f=w7848) -> (s? t:f=w7847:string)
            n3337 = call "string log (SubVI).vi"("state Name"=w7847) -> ()  [unwired: 9 in, 2 out]
          }
          frame condition #1 {
          }
        }
        n3338 = call "progress string(SubVI).vi"("String 3"=w7815, "String in"=w7816) -> ("String out"=w7817:string)  [unwired: 9 in]
        n3339 = call "FGV DRV stand.vi"() -> ("Sub-Test.DCV"=w7813:bool)  [unwired: 10 in, 1 out]
        n3340 = call "FGV Driver Data.vi"("DUT index(1-60)"=w7814) -> ("DUT SC"=w7812:bool)  [unwired: 7 in, 3 out]
        n3341 = Not(x=w7813) -> (.not. x?=w7810:bool)
        n3342 = Or(x=w7812, y=w7810) -> (x .or. y?=w7811:bool)
        n3343 = case shown="False" w7811 {
          tunnel: [w7840 _] -> w7822
          tunnel: w7819 -> [w7839 _]
          frame False {
            w7828 = T9 {"command"="", "data"=variant} ("element")
            w7827 = "MEAS.mux6_1"
            n3344 = To Variant(anything=T2."mux6_1_channel4_3" ("mux6_1(3wires)_encode")) -> (Variant=w7837:variant)
            n3345 = To Variant(anything=T2."mux6_1_channel4_2" ("mux6_1(3wires)_encode")) -> (Variant=w7835:variant)
            n3346 = Bundle By Name(cluster=w7828, "command"=w7827, "data"=w7835) -> (w7834:T9)
            n3347 = Bundle By Name(cluster=w7828, "command"=w7827, "data"=w7837) -> (w7833:T9)
            n3348 = Bundle By Name(cluster=w7828, "command"="MEAS.DMM dual read") -> (w7831:T9)
            n3349 = Build Array(w7834, w7833, w7831) -> (w7829:T9[])
            n3350 = Reverse 1D Array(array=w7829) -> (reversed array=w7830:T9[])
            n3351 = for {
              tunnel: [w7846] -> w7840 mode=indexing
              tunnel: w7839 -> [w7845]
              tunnel: w7830 -> [w7844] mode=indexing
              n3352 = Unbundle By Name(w7844) -> ("command"=w7843:string, "data"=w7842:variant)
              n3353 = call "App enquece.vi"("Priority Enquece"=TRUE, "command data"=w7842, "command"=w7843, "queue in"=w7845) -> ("error out"=w7846:errorcluster)  [unwired: 6 in, 1 out]
            }
          }
          frame True {
          }
        }
        n3354 = Merge Errors(w7820, w7822) -> (w7821:errorcluster)
      }
      frame "Test DRV 11" {
        w7855 = 11  # DUT index(1-60)
        n3355 = disable-structure shown="LOGGING==TRUE" {
          disable-tunnel: w7856 -> [w7889 _]
          frame condition #0 (active) {
            n3356 = Empty String/Path?(string/path=w7889) -> (empty?=w7891:bool)
            n3357 = Select(t="Quece timeout", s=w7891, f=w7889) -> (s? t:f=w7888:string)
            n3358 = call "string log (SubVI).vi"("state Name"=w7888) -> ()  [unwired: 9 in, 2 out]
          }
          frame condition #1 {
          }
        }
        n3359 = call "progress string(SubVI).vi"("String 3"=w7856, "String in"=w7857) -> ("String out"=w7858:string)  [unwired: 9 in]
        n3360 = call "FGV DRV stand.vi"() -> ("Sub-Test.DCV"=w7854:bool)  [unwired: 10 in, 1 out]
        n3361 = call "FGV Driver Data.vi"("DUT index(1-60)"=w7855) -> ("DUT SC"=w7853:bool)  [unwired: 7 in, 3 out]
        n3362 = Not(x=w7854) -> (.not. x?=w7851:bool)
        n3363 = Or(x=w7853, y=w7851) -> (x .or. y?=w7852:bool)
        n3364 = case shown="False" w7852 {
          tunnel: [w7881 _] -> w7863
          tunnel: w7860 -> [w7880 _]
          frame False {
            w7868 = T9 {"command"="", "data"=variant} ("element")
            w7869 = "MEAS.mux6_1"
            n3365 = To Variant(anything=T2."mux6_1_channel5_3" ("mux6_1(3wires)_encode")) -> (Variant=w7878:variant)
            n3366 = To Variant(anything=T2."mux6_1_channel5_2" ("mux6_1(3wires)_encode")) -> (Variant=w7876:variant)
            n3367 = Bundle By Name(cluster=w7868, "command"=w7869, "data"=w7876) -> (w7875:T9)
            n3368 = Bundle By Name(cluster=w7868, "command"=w7869, "data"=w7878) -> (w7874:T9)
            n3369 = Bundle By Name(cluster=w7868, "command"="MEAS.DMM dual read") -> (w7872:T9)
            n3370 = Build Array(w7875, w7874, w7872) -> (w7870:T9[])
            n3371 = Reverse 1D Array(array=w7870) -> (reversed array=w7871:T9[])
            n3372 = for {
              tunnel: [w7887] -> w7881 mode=indexing
              tunnel: w7880 -> [w7886]
              tunnel: w7871 -> [w7885] mode=indexing
              n3373 = Unbundle By Name(w7885) -> ("command"=w7884:string, "data"=w7883:variant)
              n3374 = call "App enquece.vi"("Priority Enquece"=TRUE, "command data"=w7883, "command"=w7884, "queue in"=w7886) -> ("error out"=w7887:errorcluster)  [unwired: 6 in, 1 out]
            }
          }
          frame True {
          }
        }
        n3375 = Merge Errors(w7861, w7863) -> (w7862:errorcluster)
      }
      frame "Test DRV 12" {
        w7896 = 12  # DUT index(1-60)
        n3376 = disable-structure shown="LOGGING==TRUE" {
          disable-tunnel: w7897 -> [w7930 _]
          frame condition #0 (active) {
            n3377 = Empty String/Path?(string/path=w7930) -> (empty?=w7932:bool)
            n3378 = Select(t="Quece timeout", s=w7932, f=w7930) -> (s? t:f=w7929:string)
            n3379 = call "string log (SubVI).vi"("state Name"=w7929) -> ()  [unwired: 9 in, 2 out]
          }
          frame condition #1 {
          }
        }
        n3380 = call "progress string(SubVI).vi"("String 3"=w7897, "String in"=w7898) -> ("String out"=w7899:string)  [unwired: 9 in]
        n3381 = call "FGV DRV stand.vi"() -> ("Sub-Test.DCV"=w7895:bool)  [unwired: 10 in, 1 out]
        n3382 = call "FGV Driver Data.vi"("DUT index(1-60)"=w7896) -> ("DUT SC"=w7894:bool)  [unwired: 7 in, 3 out]
        n3383 = Not(x=w7895) -> (.not. x?=w7892:bool)
        n3384 = Or(x=w7894, y=w7892) -> (x .or. y?=w7893:bool)
        n3385 = case shown="False" w7893 {
          tunnel: [w7922 _] -> w7904
          tunnel: w7901 -> [w7921 _]
          frame False {
            w7910 = T9 {"command"="", "data"=variant} ("element")
            w7909 = "MEAS.mux6_1"
            n3386 = To Variant(anything=T2."mux6_1_channel6_3" ("mux6_1(3wires)_encode")) -> (Variant=w7919:variant)
            n3387 = To Variant(anything=T2."mux6_1_channel6_2" ("mux6_1(3wires)_encode")) -> (Variant=w7917:variant)
            n3388 = Bundle By Name(cluster=w7910, "command"=w7909, "data"=w7917) -> (w7916:T9)
            n3389 = Bundle By Name(cluster=w7910, "command"=w7909, "data"=w7919) -> (w7915:T9)
            n3390 = Bundle By Name(cluster=w7910, "command"="MEAS.DMM dual read") -> (w7913:T9)
            n3391 = Build Array(w7916, w7915, w7913) -> (w7911:T9[])
            n3392 = Reverse 1D Array(array=w7911) -> (reversed array=w7912:T9[])
            n3393 = for {
              tunnel: [w7928] -> w7922 mode=indexing
              tunnel: w7921 -> [w7927]
              tunnel: w7912 -> [w7926] mode=indexing
              n3394 = Unbundle By Name(w7926) -> ("command"=w7925:string, "data"=w7924:variant)
              n3395 = call "App enquece.vi"("Priority Enquece"=TRUE, "command data"=w7924, "command"=w7925, "queue in"=w7927) -> ("error out"=w7928:errorcluster)  [unwired: 6 in, 1 out]
            }
          }
          frame True {
          }
        }
        n3396 = Merge Errors(w7902, w7904) -> (w7903:errorcluster)
      }
      frame "Test DRV 13" {
        w7937 = 13  # DUT index(1-60)
        n3397 = call "progress string(SubVI).vi"("String 3"=w7938, "String in"=w7939) -> ("String out"=w7940:string)  [unwired: 9 in]
        n3398 = disable-structure shown="LOGGING==TRUE" {
          disable-tunnel: w7938 -> [w7971 _]
          frame condition #0 (active) {
            n3399 = Empty String/Path?(string/path=w7971) -> (empty?=w7973:bool)
            n3400 = Select(t="Quece timeout", s=w7973, f=w7971) -> (s? t:f=w7970:string)
            n3401 = call "string log (SubVI).vi"("state Name"=w7970) -> ()  [unwired: 9 in, 2 out]
          }
          frame condition #1 {
          }
        }
        n3402 = call "FGV DRV stand.vi"() -> ("Sub-Test.DCV"=w7936:bool)  [unwired: 10 in, 1 out]
        n3403 = Not(x=w7936) -> (.not. x?=w7933:bool)
        n3404 = call "FGV Driver Data.vi"("DUT index(1-60)"=w7937) -> ("DUT SC"=w7935:bool)  [unwired: 7 in, 3 out]
        n3405 = Or(x=w7935, y=w7933) -> (x .or. y?=w7934:bool)
        n3406 = case shown="True" w7934 {
          tunnel: [w7963 _] -> w7945
          tunnel: w7942 -> [w7962 _]
          frame False {
            w7951 = T9 {"command"="", "data"=variant} ("element")
            w7950 = "MEAS.mux6_1"
            n3407 = To Variant(anything=T2."mux6_1_channel1_3" ("mux6_1(3wires)_encode")) -> (Variant=w7960:variant)
            n3408 = To Variant(anything=T2."mux6-1_channel1_2" ("mux6_1(3wires)_encode")) -> (Variant=w7958:variant)
            n3409 = Bundle By Name(cluster=w7951, "command"=w7950, "data"=w7958) -> (w7957:T9)
            n3410 = Bundle By Name(cluster=w7951, "command"=w7950, "data"=w7960) -> (w7956:T9)
            n3411 = Bundle By Name(cluster=w7951, "command"="MEAS.DMM dual read") -> (w7954:T9)
            n3412 = Build Array(w7957, w7956, w7954) -> (w7952:T9[])
            n3413 = Reverse 1D Array(array=w7952) -> (reversed array=w7953:T9[])
            n3414 = for {
              tunnel: [w7969] -> w7963 mode=indexing
              tunnel: w7962 -> [w7968]
              tunnel: w7953 -> [w7967] mode=indexing
              n3415 = Unbundle By Name(w7967) -> ("command"=w7966:string, "data"=w7965:variant)
              n3416 = call "App enquece.vi"("Priority Enquece"=TRUE, "command data"=w7965, "command"=w7966, "queue in"=w7968) -> ("error out"=w7969:errorcluster)  [unwired: 6 in, 1 out]
            }
          }
          frame True {
          }
        }
        n3417 = Merge Errors(w7943, w7945) -> (w7944:errorcluster)
      }
      frame "Test DRV 14" {
        w7978 = 14  # DUT index(1-60)
        n3418 = disable-structure shown="LOGGING==TRUE" {
          disable-tunnel: w7979 -> [w8012 _]
          frame condition #0 (active) {
            n3419 = Empty String/Path?(string/path=w8012) -> (empty?=w8014:bool)
            n3420 = Select(t="Quece timeout", s=w8014, f=w8012) -> (s? t:f=w8011:string)
            n3421 = call "string log (SubVI).vi"("state Name"=w8011) -> ()  [unwired: 9 in, 2 out]
          }
          frame condition #1 {
          }
        }
        n3422 = call "progress string(SubVI).vi"("String 3"=w7979, "String in"=w7980) -> ("String out"=w7981:string)  [unwired: 9 in]
        n3423 = call "FGV DRV stand.vi"() -> ("Sub-Test.DCV"=w7977:bool)  [unwired: 10 in, 1 out]
        n3424 = call "FGV Driver Data.vi"("DUT index(1-60)"=w7978) -> ("DUT SC"=w7976:bool)  [unwired: 7 in, 3 out]
        n3425 = Not(x=w7977) -> (.not. x?=w7974:bool)
        n3426 = Or(x=w7976, y=w7974) -> (x .or. y?=w7975:bool)
        n3427 = case shown="False" w7975 {
          tunnel: [w8004 _] -> w7986
          tunnel: w7983 -> [w8003 _]
          frame False {
            w7992 = T9 {"command"="", "data"=variant} ("element")
            w7991 = "MEAS.mux6_1"
            n3428 = To Variant(anything=T2."mux6_1_channel2_3" ("mux6_1(3wires)_encode")) -> (Variant=w8001:variant)
            n3429 = To Variant(anything=T2."mux6_1_channel2_2" ("mux6_1(3wires)_encode")) -> (Variant=w7999:variant)
            n3430 = Bundle By Name(cluster=w7992, "command"=w7991, "data"=w7999) -> (w7998:T9)
            n3431 = Bundle By Name(cluster=w7992, "command"=w7991, "data"=w8001) -> (w7997:T9)
            n3432 = Bundle By Name(cluster=w7992, "command"="MEAS.DMM dual read") -> (w7995:T9)
            n3433 = Build Array(w7998, w7997, w7995) -> (w7993:T9[])
            n3434 = Reverse 1D Array(array=w7993) -> (reversed array=w7994:T9[])
            n3435 = for {
              tunnel: [w8010] -> w8004 mode=indexing
              tunnel: w8003 -> [w8009]
              tunnel: w7994 -> [w8008] mode=indexing
              n3436 = Unbundle By Name(w8008) -> ("command"=w8007:string, "data"=w8006:variant)
              n3437 = call "App enquece.vi"("Priority Enquece"=TRUE, "command data"=w8006, "command"=w8007, "queue in"=w8009) -> ("error out"=w8010:errorcluster)  [unwired: 6 in, 1 out]
            }
          }
          frame True {
          }
        }
        n3438 = Merge Errors(w7984, w7986) -> (w7985:errorcluster)
      }
      frame "Test DRV 15" {
        w8019 = 15  # DUT index(1-60)
        n3439 = disable-structure shown="LOGGING==TRUE" {
          disable-tunnel: w8020 -> [w8053 _]
          frame condition #0 (active) {
            n3440 = Empty String/Path?(string/path=w8053) -> (empty?=w8055:bool)
            n3441 = Select(t="Quece timeout", s=w8055, f=w8053) -> (s? t:f=w8052:string)
            n3442 = call "string log (SubVI).vi"("state Name"=w8052) -> ()  [unwired: 9 in, 2 out]
          }
          frame condition #1 {
          }
        }
        n3443 = call "progress string(SubVI).vi"("String 3"=w8020, "String in"=w8021) -> ("String out"=w8022:string)  [unwired: 9 in]
        n3444 = call "FGV DRV stand.vi"() -> ("Sub-Test.DCV"=w8018:bool)  [unwired: 10 in, 1 out]
        n3445 = call "FGV Driver Data.vi"("DUT index(1-60)"=w8019) -> ("DUT SC"=w8017:bool)  [unwired: 7 in, 3 out]
